vi "Flush.vi"(11 "POTTypedCircularBuffer in":refnum<class "POTTypedCircularBuffer.lvclass">) -> (3 "POTTypedCircularBuffer out":refnum<class "POTTypedCircularBuffer.lvclass">)   [LabVIEW 2024, in "POTTypedCircularBuffer.lvclass"]
uses:
  POTTypedCircularBuffer.lvclass
  POTTypedCircularBuffer.lvclass/POTTypedCircularBuffer.ctl
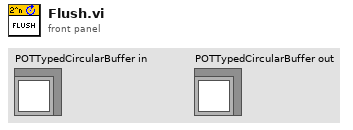
[diagram p1: front panel]
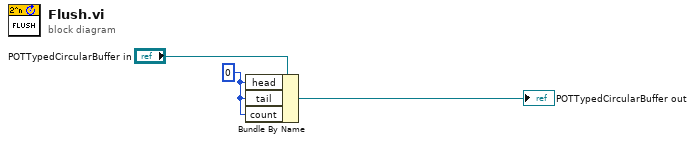
[diagram p0: block diagram]
diagram:
  w1 = 0 ("head")
  n1 = Bundle By Name(cluster="POTTypedCircularBuffer in", "head"=w1, "tail"=w1, "count"=w1) -> (→"POTTypedCircularBuffer out":refnum<class "POTTypedCircularBuffer.lvclass">)
